vi "Deadband.vi"(10 "Deadband":dbl, 11 "Robot Velocities":T1) -> (2 "Sending Input?":bool, 3 "Adjusted Robot Velocities":T1)   [LabVIEW 2020]
uses:
  swerve/Type Definitions/Data/Robot Velocities.ctl
  <vilib>/Analysis/_algsub.llb/Real Vector Norm.vi
  <vilib>/Analysis/NI_AALPro.lvlib
panel:
  in  "New High":dbl
  in  "New Low":dbl
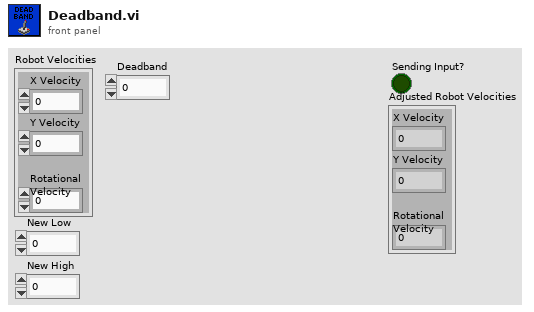
[diagram p1: front panel]
types:
  T1 = typedef "Robot Velocities.ctl" = cluster{"X Velocity":dbl, "Y Velocity":dbl, "Rotational \nVelocity":dbl}
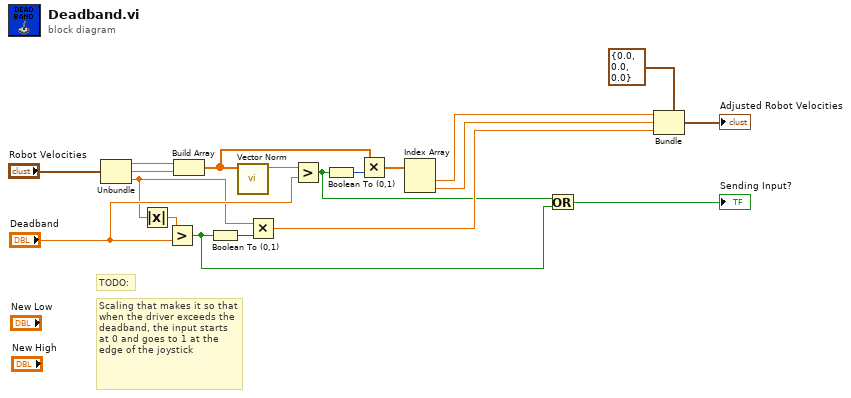
[diagram p0: block diagram]
diagram:
  # "TODO:"
  # "Scaling that makes it so that when the driver exceeds the deadband, the input starts at 0 and goes to 1 at the edge of the joystick"
  n1 = Unbundle("Robot Velocities") -> ("X Velocity"=w18:dbl, "Y Velocity"=w17:dbl, "Rotational \nVelocity"=w2:dbl)
  n2 = Absolute Value(x=w2) -> (abs(x)=w1:dbl)
  n3 = Greater?(x=w1, y="Deadband") -> (0:w15:bool)
  n4 = Build Array(w18, w17) -> (w10:dbl[])
  n5 = Boolean To (0,1)(Boolean=w15) -> (0, 1=w16:i16)
  n6 = call-poly <vilib>:"Vector Norm.vi"("Input Vector"=w10) -> ("norm"=w12:dbl)  [unwired: 9 in, 1 out]
  n7 = Multiply(x=w2, y=w16) -> (x*y=w5:dbl)
  n8 = Greater?(x=w12, y="Deadband") -> (0:w4:bool)
  n9 = Boolean To (0,1)(Boolean=w4) -> (0, 1=w11:i16)
  n10 = Multiply(x=w10, y=w11) -> (x*y=w8:dbl[])
  n11 = Index Array(array=w8) -> (element #1=w7:dbl, element #2=w6:dbl)  [unwired: 2 in]
  n12 = Or(x=w4, y=w15) -> (x .or. y?=→"Sending Input?":bool)
  n13 = Bundle(cluster=T1 {"X Velocity"=0.0, "Y Velocity"=0.0, "Rotational \nVelocity"=0.0} ("Adjusted Robot Velocities"), "X Velocity"=w7, "Y Velocity"=w6, "Rotational \nVelocity"=w5) -> (→"Adjusted Robot Velocities":T1)
